vi "Column Property Node.vi"   [LabVIEW 2023, in "SQLiteSupport.lvlib"]
uses:
  SQLiteSupport.lvlib
  SQL Statement.lvclass
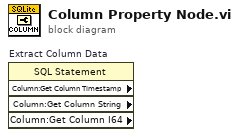
[diagram p0: block diagram]
diagram:
  n1 = property on="Extract Column Data" class="SQL Statement" props=["Column:Get Column Timestamp", "Column:Get Column String", "Column:Get Column I64"]() -> ()  [unwired: 2 in, 5 out]
